vi "SET_SUPPLY_n.vi"(2 "execute":bool, 7 "supply":bool, 11 "error in (no error)":errorcluster) -> (4 "function return":string, 15 "error out":errorcluster)   [LabVIEW 2017, in "ZBOX_IS.lvlib"]
uses:
  ZBOX_IS.lvlib
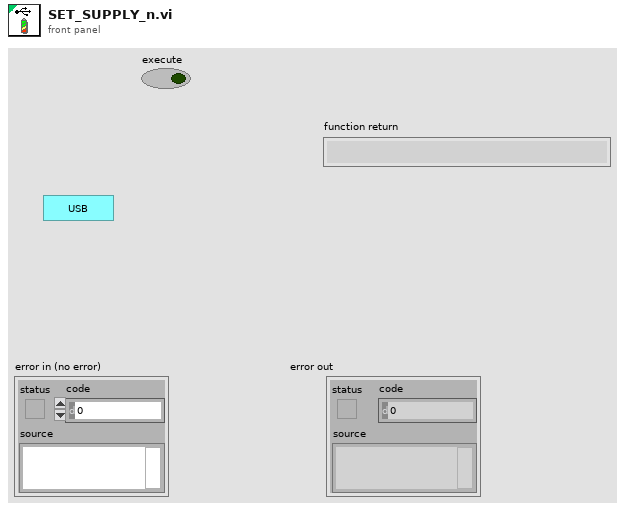
[diagram p1: front panel]
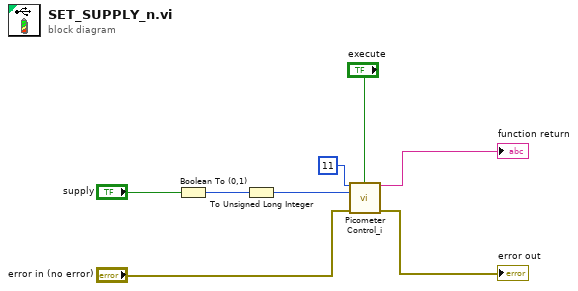
[diagram p0: block diagram]
diagram:
  n1 = Boolean To (0,1)(Boolean="supply") -> (0, 1=w3:i16)
  n2 = To Unsigned Long Integer(number=w3) -> (unsigned 32bit integer=w2:u32)
  n3 = call "Picometer Control_i.vi"("Cmd"=u8 11, "execute"="execute", "ulValue"=w2, "error in (no error)"="error in (no error)") -> ("function return"=→"function return":string, "error out"=→"error out":errorcluster)  [unwired: 7 in, 3 out]
